vi "CONEX_FUNCTIONAL_GLOBAL.vi"(6 "Axis":enum16{"X", "Y", "Z", "XY", "XZ", "YZ", "XYZ"}(ring), 8 "error in":errorcluster, 9 "ASCII command":string, 10 "Position":dbl[](array[numeric]), 11 "Command":T1(ring)) -> (0 "error out":errorcluster, 1 "ASCII response":string[](array[string]), 2 "Current Position":dbl[](array[numeric]))   [LabVIEW 2013]
uses:
  <vilib>/Instr/_visa.llb/VISA Flush IO Buffer Mask.ctl
  <vilib>/Instr/_visa.llb/VISA Configure Serial Port (Instr).vi
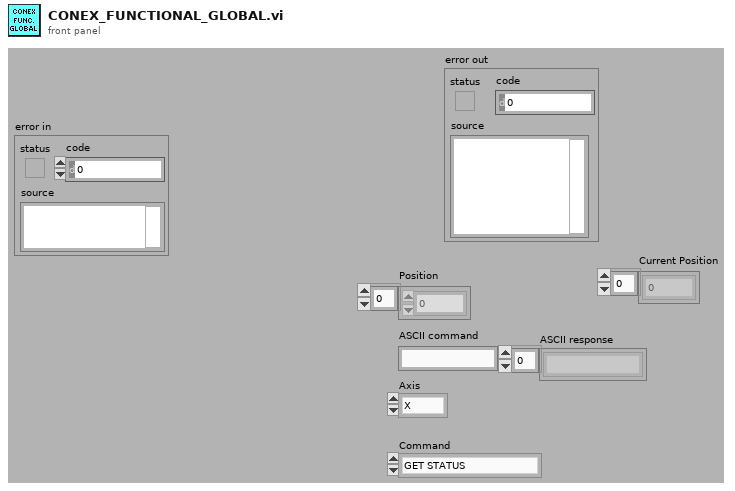
[diagram p1: front panel]
types:
  T1 = enum16{"GET STATUS", "ABS MOVE", "GET POS", "REL MOVE", "INIT", "CLOSE", "HOME", "READ ASCII", "ASCII", "SET ULIM", "STOP", "SET LLIM"}
  T2 = typedef "VISA Flush IO Buffer Mask.ctl" = u16
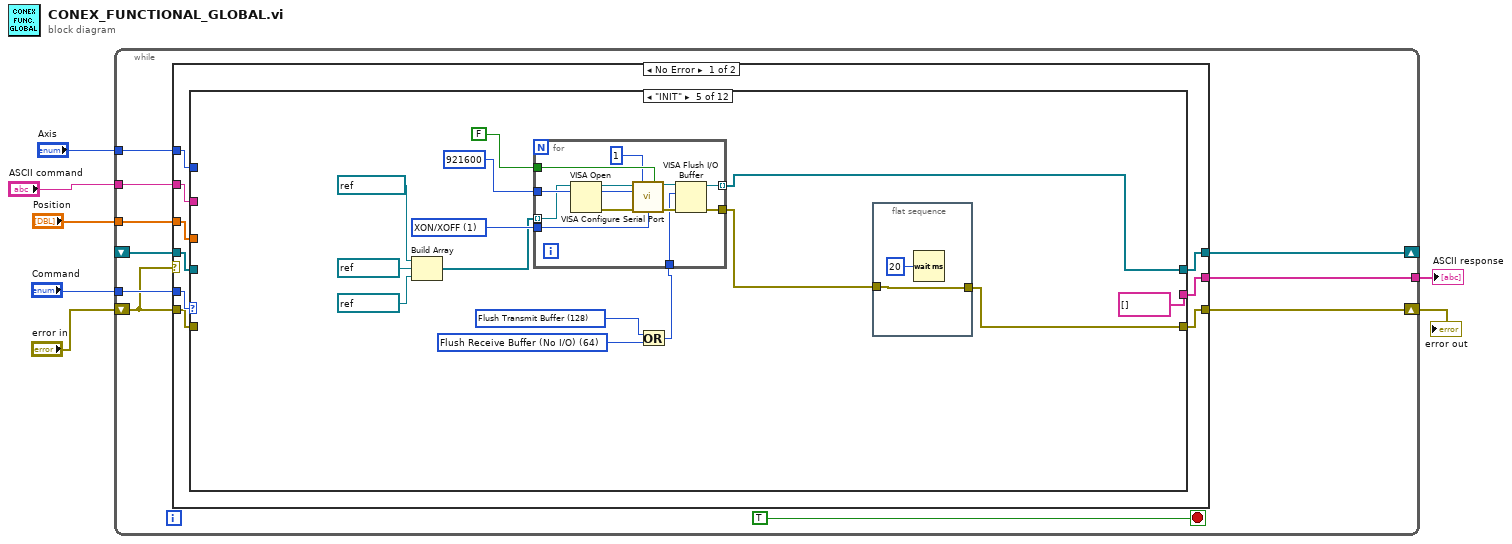
[diagram p0: block diagram]
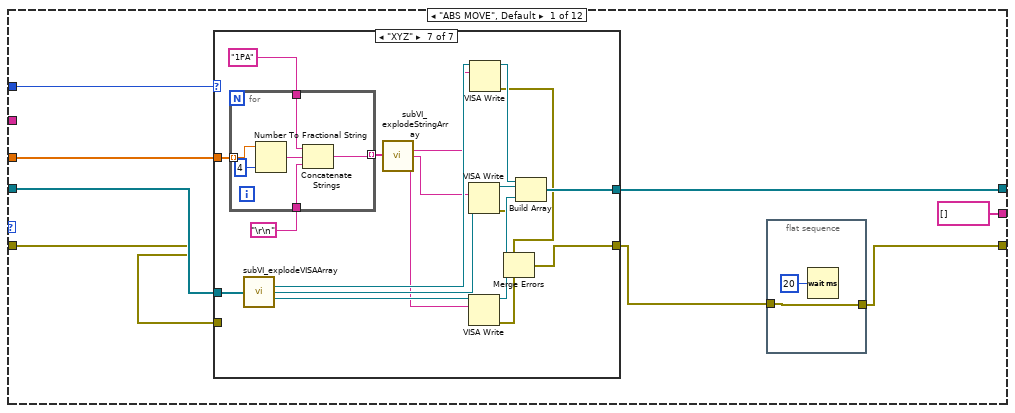
[diagram p2: hidden frame]
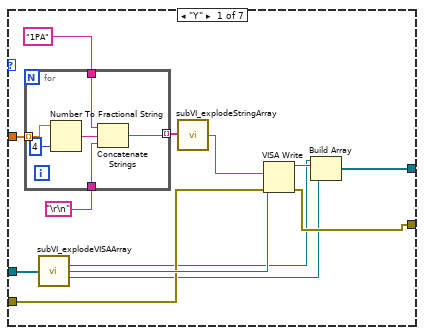
[diagram p3: hidden frame]
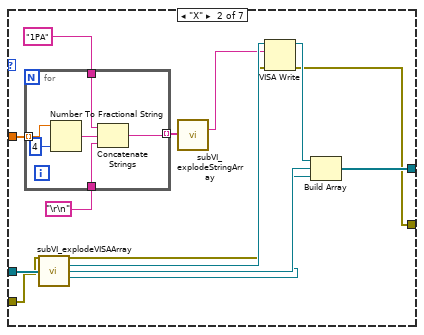
[diagram p4: hidden frame]
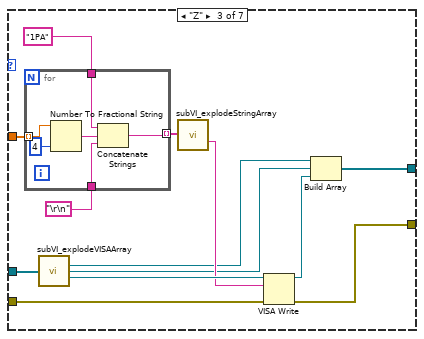
[diagram p5: hidden frame]
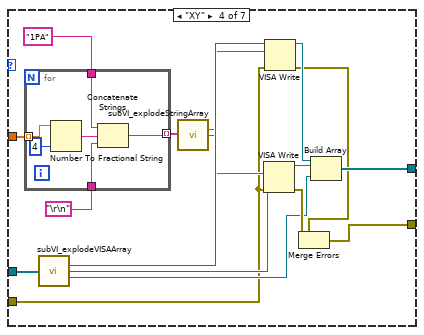
[diagram p6: hidden frame]
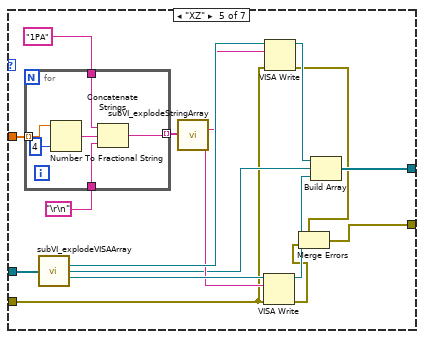
[diagram p7: hidden frame]
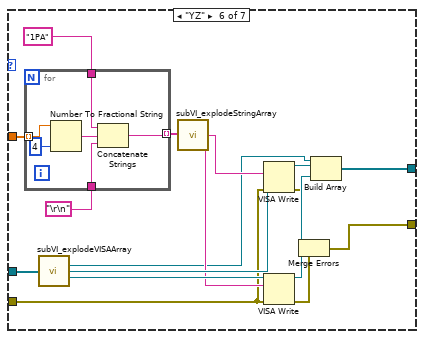
[diagram p8: hidden frame]
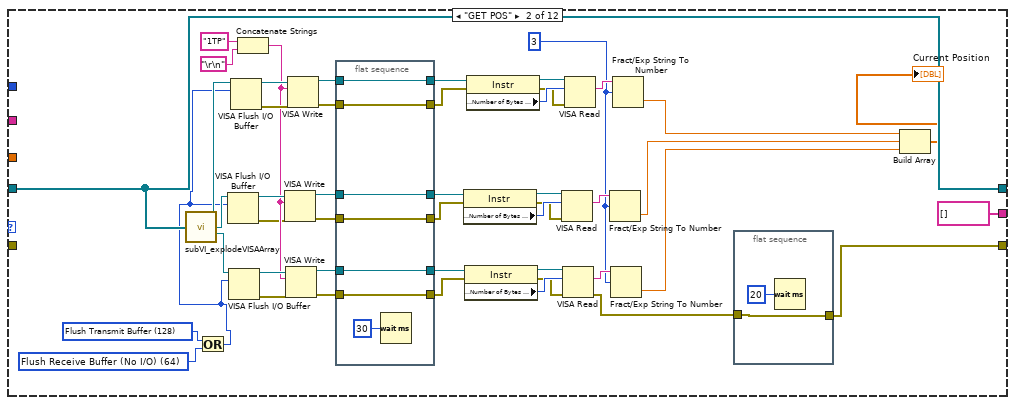
[diagram p9: hidden frame]
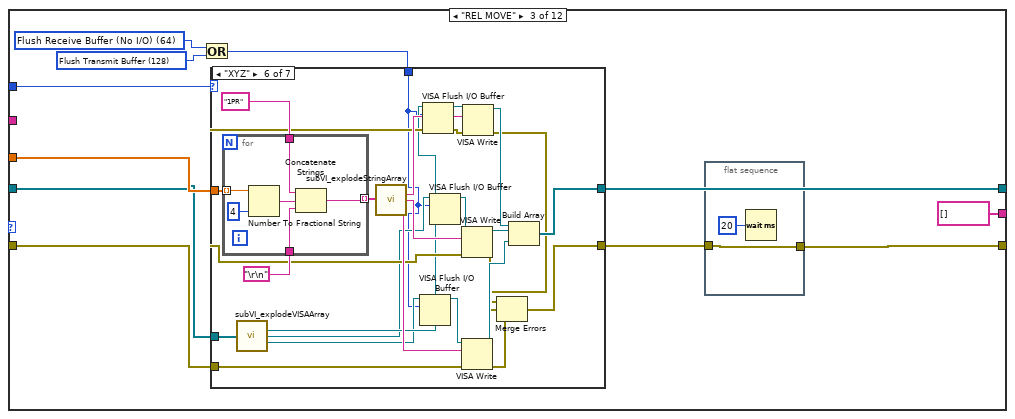
[diagram p10: hidden frame]
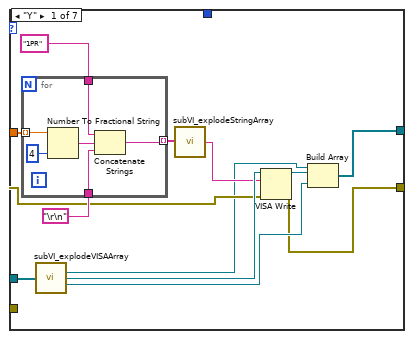
[diagram p11: hidden frame]
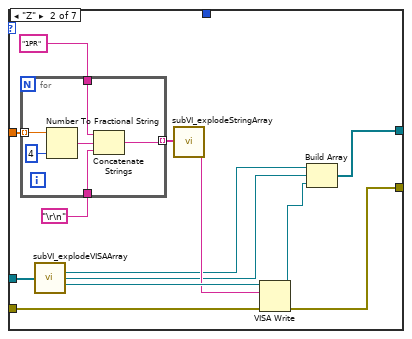
[diagram p12: hidden frame]
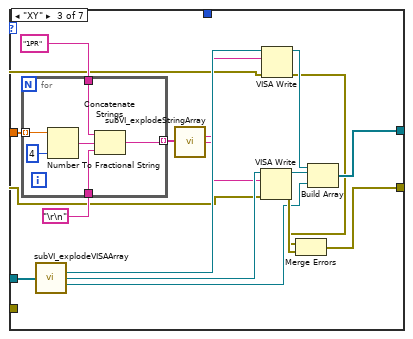
[diagram p13: hidden frame]
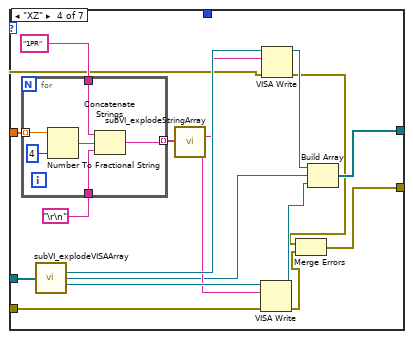
[diagram p14: hidden frame]
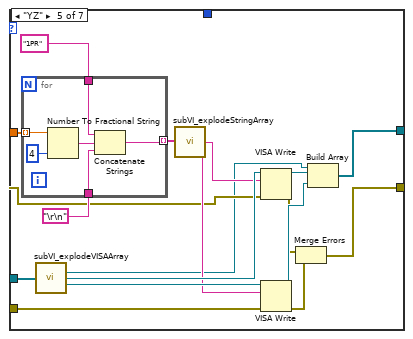
[diagram p15: hidden frame]
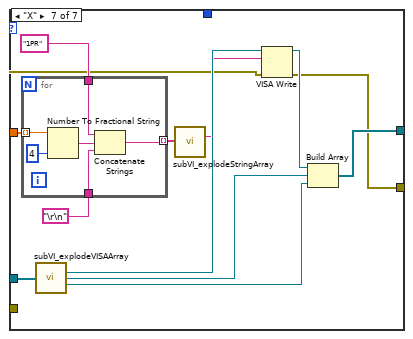
[diagram p16: hidden frame]
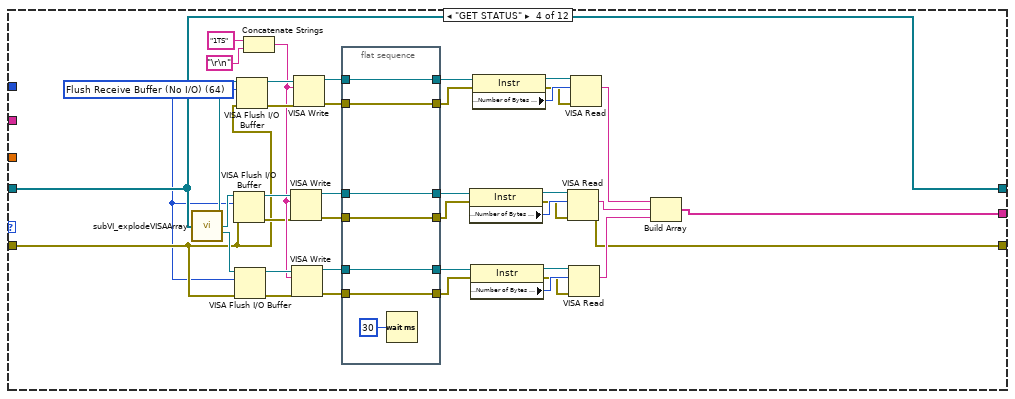
[diagram p17: hidden frame]
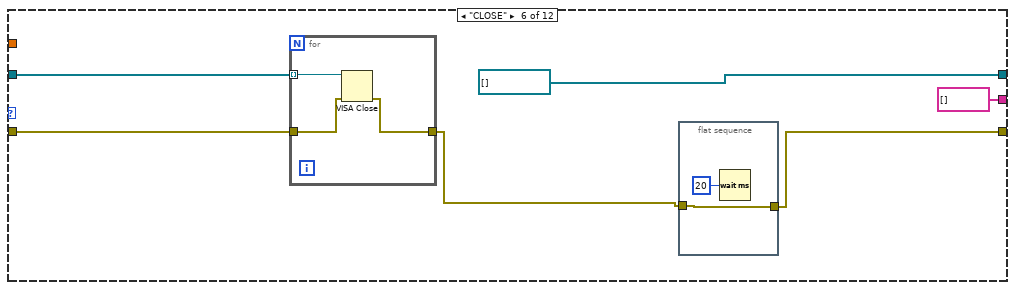
[diagram p18: hidden frame]
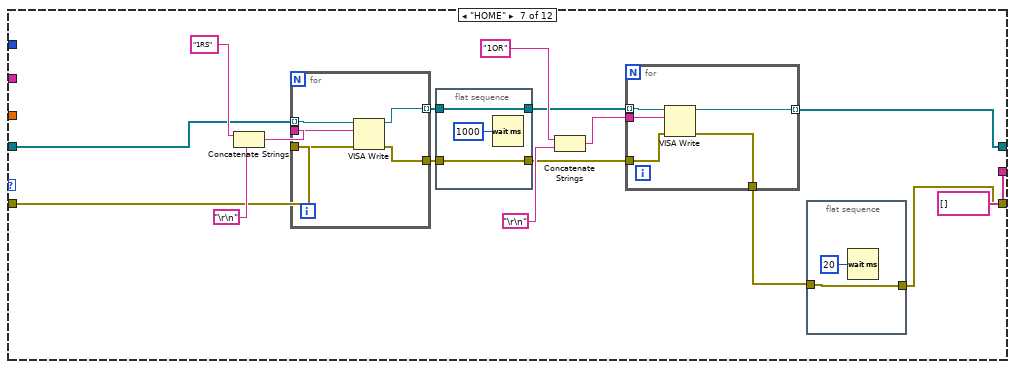
[diagram p19: hidden frame]
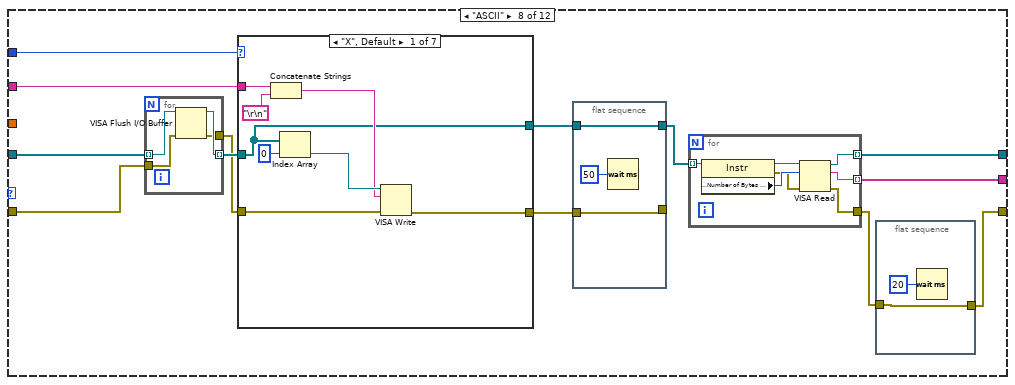
[diagram p20: hidden frame]
diagram:
  n1 = while {
    tunnel: "Command" -> [w17]
    shift-right: [w16] -> _
    shift-left: _ -> [w14]
    shift-right: [w15] -> w3
    shift-left: "error in" -> [w8]
    tunnel: "Position" -> [w13]
    tunnel: "ASCII command" -> [w11]
    tunnel: "Axis" -> [w10]
    tunnel: [w9] -> w1
    stop <- TRUE stop-if-true
    n2 = case shown="No Error" w8 {
      tunnel: w17 -> [w26 _]
      tunnel: [w25 refnum<visa-resource-name>[] []] -> w16
      tunnel: [w24 errorcluster {"status"=FALSE, "code"=0, "source"=""} ("error out")] -> w15
      tunnel: w14 -> [w23 w812]
      tunnel: w8 -> [w22 w811]
      tunnel: w13 -> [w21 _]
      tunnel: w11 -> [w20 _]
      tunnel: w10 -> [w19 _]
      tunnel: [w18 string[] []] -> w9
      frame No Error {
        n3 = case shown="\"INIT\"" w26 {
          tunnel: [w32 w232 w252 w417 w474 refnum<visa-resource-name>[] [] w513 w535 w638 w653 w671 w690] -> w25
          tunnel: [w27 w188 w245 w415 w462 w490 w501 w532 w635 w651 w669 w687] -> w24
          tunnel: w23 -> [w34 w232 w253 w417 _ w495 w509 w540 w643 w654 w672 w693]
          tunnel: w22 -> [w30 _ w254 w416 _ w494 w508 w538 w639 w657 w675 w692]
          tunnel: w21 -> [w33 _ w255 _ _ _ _ _ _ w655 w673 _]
          tunnel: w20 -> [_ _ _ _ _ _ _ w543 _ _ _ w694]
          tunnel: w19 -> [w31 _ w251 _ _ _ _ w544 _ _ _ w691]
          tunnel: [string[] [] string[] [] string[] [] w418 string[] [] string[] [] string[] [] w534 string[] [] string[] [] string[] [] w689] -> w18
          frame "ABS MOVE", Default {
            n4 = case shown="\"XYZ\"" w31 {
              tunnel: w34 -> [w49 w68 w87 w110 w133 w156 w181]
              tunnel: w33 -> [w47 w66 w85 w107 w130 w153 w177]
              tunnel: [w41 w60 w79 w99 w122 w145 w167] -> w32
              tunnel: [w40 w57 w76 w96 w120 w142 w163] -> w28
              tunnel: w30 -> [w39 w56 w75 w94 w118 w140 _]
              frame "Y" {
                n5 = for {
                  tunnel: w47 -> [w55] mode=indexing
                  tunnel: "1PA" -> [w53]
                  tunnel: "\r\n" -> [w52]
                  tunnel: [w51] -> w44 mode=indexing
                  n6 = Number To Fractional String(number=w55, precision (6)=i16 4) -> (F-format string=w54:string)  [unwired: 2 in]
                  n7 = Concatenate Strings(w53, w54, w52) -> (w51:string)
                }
                n8 = call "subVI_explodeVISAArray.vi"("Array"=w49) -> ("x"=w38:refnum<visa-resource-name>, "y"=w48:refnum<visa-resource-name>, "z"=w37:refnum<visa-resource-name>)  [unwired: 12 in]
                n9 = call "subVI_explodeStringArray.vi"("Array"=w44) -> ("y"=w43:string)  [unwired: 12 in, 2 out]
                n10 = VISA Write(VISA resource name=w48, write buffer=w43, error in (no error)=w39) -> (VISA resource name out=w42:refnum<visa-resource-name>, error out=w40:errorcluster)  [unwired: 1 out]
                n11 = Build Array(w38, w42, w37) -> (w41:refnum<visa-resource-name>[])
              }
              frame "X" {
                n12 = for {
                  tunnel: w66 -> [w74] mode=indexing
                  tunnel: "1PA" -> [w72]
                  tunnel: "\r\n" -> [w71]
                  tunnel: [w70] -> w63 mode=indexing
                  n13 = Number To Fractional String(number=w74, precision (6)=i16 4) -> (F-format string=w73:string)  [unwired: 2 in]
                  n14 = Concatenate Strings(w72, w73, w71) -> (w70:string)
                }
                n15 = call "subVI_explodeVISAArray.vi"("Array"=w68) -> ("x"=w67:refnum<visa-resource-name>, "y"=w59:refnum<visa-resource-name>, "z"=w58:refnum<visa-resource-name>)  [unwired: 12 in]
                n16 = call "subVI_explodeStringArray.vi"("Array"=w63) -> ("x"=w62:string)  [unwired: 12 in, 2 out]
                n17 = VISA Write(VISA resource name=w67, write buffer=w62, error in (no error)=w56) -> (VISA resource name out=w61:refnum<visa-resource-name>, error out=w57:errorcluster)  [unwired: 1 out]
                n18 = Build Array(w61, w59, w58) -> (w60:refnum<visa-resource-name>[])
              }
              frame "Z" {
                n19 = for {
                  tunnel: w85 -> [w93] mode=indexing
                  tunnel: "1PA" -> [w91]
                  tunnel: "\r\n" -> [w90]
                  tunnel: [w89] -> w82 mode=indexing
                  n20 = Number To Fractional String(number=w93, precision (6)=i16 4) -> (F-format string=w92:string)  [unwired: 2 in]
                  n21 = Concatenate Strings(w91, w92, w90) -> (w89:string)
                }
                n22 = call "subVI_explodeVISAArray.vi"("Array"=w87) -> ("x"=w78:refnum<visa-resource-name>, "y"=w77:refnum<visa-resource-name>, "z"=w86:refnum<visa-resource-name>)  [unwired: 12 in]
                n23 = call "subVI_explodeStringArray.vi"("Array"=w82) -> ("z"=w81:string)  [unwired: 12 in, 2 out]
                n24 = VISA Write(VISA resource name=w86, write buffer=w81, error in (no error)=w75) -> (VISA resource name out=w80:refnum<visa-resource-name>, error out=w76:errorcluster)  [unwired: 1 out]
                n25 = Build Array(w78, w77, w80) -> (w79:refnum<visa-resource-name>[])
              }
              frame "XY" {
                n26 = for {
                  tunnel: w107 -> [w116] mode=indexing
                  tunnel: "1PA" -> [w114]
                  tunnel: "\r\n" -> [w113]
                  tunnel: [w112] -> w104 mode=indexing
                  n27 = Number To Fractional String(number=w116, precision (6)=i16 4) -> (F-format string=w115:string)  [unwired: 2 in]
                  n28 = Concatenate Strings(w114, w115, w113) -> (w112:string)
                }
                n29 = call "subVI_explodeVISAArray.vi"("Array"=w110) -> ("x"=w109:refnum<visa-resource-name>, "y"=w108:refnum<visa-resource-name>, "z"=w95:refnum<visa-resource-name>)  [unwired: 12 in]
                n30 = call "subVI_explodeStringArray.vi"("Array"=w104) -> ("x"=w103:string, "y"=w102:string)  [unwired: 12 in, 1 out]
                n31 = VISA Write(VISA resource name=w108, write buffer=w102, error in (no error)=w94) -> (VISA resource name out=w100:refnum<visa-resource-name>, error out=w97:errorcluster)  [unwired: 1 out]
                n32 = VISA Write(VISA resource name=w109, write buffer=w103, error in (no error)=w94) -> (VISA resource name out=w101:refnum<visa-resource-name>, error out=w98:errorcluster)  [unwired: 1 out]
                n33 = Merge Errors(w98, w97) -> (w96:errorcluster)
                n34 = Build Array(w101, w100, w95) -> (w99:refnum<visa-resource-name>[])
              }
              frame "XZ" {
                n35 = for {
                  tunnel: w130 -> [w139] mode=indexing
                  tunnel: "1PA" -> [w137]
                  tunnel: "\r\n" -> [w136]
                  tunnel: [w135] -> w127 mode=indexing
                  n36 = Number To Fractional String(number=w139, precision (6)=i16 4) -> (F-format string=w138:string)  [unwired: 2 in]
                  n37 = Concatenate Strings(w137, w138, w136) -> (w135:string)
                }
                n38 = call "subVI_explodeVISAArray.vi"("Array"=w133) -> ("x"=w132:refnum<visa-resource-name>, "y"=w119:refnum<visa-resource-name>, "z"=w131:refnum<visa-resource-name>)  [unwired: 12 in]
                n39 = call "subVI_explodeStringArray.vi"("Array"=w127) -> ("x"=w126:string, "z"=w125:string)  [unwired: 12 in, 1 out]
                n40 = VISA Write(VISA resource name=w131, write buffer=w125, error in (no error)=w118) -> (VISA resource name out=w123:refnum<visa-resource-name>, error out=w117:errorcluster)  [unwired: 1 out]
                n41 = VISA Write(VISA resource name=w132, write buffer=w126, error in (no error)=w118) -> (VISA resource name out=w124:refnum<visa-resource-name>, error out=w121:errorcluster)  [unwired: 1 out]
                n42 = Merge Errors(w121, w117) -> (w120:errorcluster)
                n43 = Build Array(w124, w119, w123) -> (w122:refnum<visa-resource-name>[])
              }
              frame "YZ" {
                n44 = for {
                  tunnel: w153 -> [w162] mode=indexing
                  tunnel: "1PA" -> [w160]
                  tunnel: "\r\n" -> [w159]
                  tunnel: [w158] -> w150 mode=indexing
                  n45 = Number To Fractional String(number=w162, precision (6)=i16 4) -> (F-format string=w161:string)  [unwired: 2 in]
                  n46 = Concatenate Strings(w160, w161, w159) -> (w158:string)
                }
                n47 = call "subVI_explodeVISAArray.vi"("Array"=w156) -> ("x"=w141:refnum<visa-resource-name>, "y"=w155:refnum<visa-resource-name>, "z"=w154:refnum<visa-resource-name>)  [unwired: 12 in]
                n48 = call "subVI_explodeStringArray.vi"("Array"=w150) -> ("y"=w149:string, "z"=w148:string)  [unwired: 12 in, 1 out]
                n49 = VISA Write(VISA resource name=w155, write buffer=w149, error in (no error)=w140) -> (VISA resource name out=w146:refnum<visa-resource-name>, error out=w144:errorcluster)  [unwired: 1 out]
                n50 = VISA Write(VISA resource name=w154, write buffer=w148, error in (no error)=w140) -> (VISA resource name out=w147:refnum<visa-resource-name>, error out=w143:errorcluster)  [unwired: 1 out]
                n51 = Merge Errors(w144, w143) -> (w142:errorcluster)
                n52 = Build Array(w141, w146, w147) -> (w145:refnum<visa-resource-name>[])
              }
              frame "XYZ" {
                n53 = for {
                  tunnel: w177 -> [w187] mode=indexing
                  tunnel: "1PA" -> [w185]
                  tunnel: "\r\n" -> [w184]
                  tunnel: [w183] -> w174 mode=indexing
                  n54 = Number To Fractional String(number=w187, precision (6)=i16 4) -> (F-format string=w186:string)  [unwired: 2 in]
                  n55 = Concatenate Strings(w185, w186, w184) -> (w183:string)
                }
                n56 = call "subVI_explodeVISAArray.vi"("Array"=w181) -> ("x"=w180:refnum<visa-resource-name>, "y"=w179:refnum<visa-resource-name>, "z"=w178:refnum<visa-resource-name>)  [unwired: 12 in]
                n57 = call "subVI_explodeStringArray.vi"("Array"=w174) -> ("x"=w173:string, "y"=w172:string, "z"=w171:string)  [unwired: 12 in]
                n58 = VISA Write(VISA resource name=w179, write buffer=w172) -> (VISA resource name out=w168:refnum<visa-resource-name>, error out=w165:errorcluster)  [unwired: 1 in, 1 out]
                n59 = VISA Write(VISA resource name=w178, write buffer=w171) -> (VISA resource name out=w169:refnum<visa-resource-name>, error out=w164:errorcluster)  [unwired: 1 in, 1 out]
                n60 = VISA Write(VISA resource name=w180, write buffer=w173) -> (VISA resource name out=w170:refnum<visa-resource-name>, error out=w166:errorcluster)  [unwired: 1 in, 1 out]
                n61 = Merge Errors(w166, w165, w164) -> (w163:errorcluster)
                n62 = Build Array(w170, w168, w169) -> (w167:refnum<visa-resource-name>[])
              }
            }
            n63 = flat-sequence {
              tunnel: w28 -> [w36]
              tunnel: [w36] -> w27
              frame #0 {
                n64 = Wait (ms)(milliseconds to wait=u32 20) -> ()  [unwired: 1 out]
              }
            }
          }
          frame "GET POS" {
            w191 = T2 64 items=["Flush Receive Buffer"=16, "Write Transmit Buffer to Device"=32, "Flush Receive Buffer (No I/O)"=64, "Flush Transmit Buffer"=128] ("Mask")
            w192 = T2 128 items=["Flush Receive Buffer"=16, "Write Transmit Buffer to Device"=32, "Flush Receive Buffer (No I/O)"=64, "Flush Transmit Buffer"=128] ("Mask")
            w195 = 3 ("offset")
            n65 = call "subVI_explodeVISAArray.vi"("Array"=w232) -> ("x"=w230:refnum<visa-resource-name>, "y"=w220:refnum<visa-resource-name>, "z"=w218:refnum<visa-resource-name>)  [unwired: 12 in]
            n66 = Or(x=w192, y=w191) -> (x .or. y?=w190:T2)
            n67 = VISA Flush I/O Buffer(VISA resource name=w220, mask (16)=w190) -> (VISA resource name out=w219:refnum<visa-resource-name>, error out=w214:errorcluster)  [unwired: 1 in]
            n68 = VISA Flush I/O Buffer(VISA resource name=w218, mask (16)=w190) -> (VISA resource name out=w217:refnum<visa-resource-name>, error out=w215:errorcluster)  [unwired: 1 in]
            n69 = VISA Flush I/O Buffer(VISA resource name=w230, mask (16)=w190) -> (VISA resource name out=w228:refnum<visa-resource-name>, error out=w229:errorcluster)  [unwired: 1 in]
            n70 = Concatenate Strings("1TP" ("string"), "\r\n") -> (w216:string)
            n71 = VISA Write(VISA resource name=w219, write buffer=w216, error in (no error)=w214) -> (VISA resource name out=w213:refnum<visa-resource-name>, error out=w210:errorcluster)  [unwired: 1 out]
            n72 = VISA Write(VISA resource name=w217, write buffer=w216, error in (no error)=w215) -> (VISA resource name out=w212:refnum<visa-resource-name>, error out=w211:errorcluster)  [unwired: 1 out]
            n73 = VISA Write(VISA resource name=w228, write buffer=w216, error in (no error)=w229) -> (VISA resource name out=w227:refnum<visa-resource-name>, error out=w226:errorcluster)  [unwired: 1 out]
            n74 = flat-sequence {
              tunnel: w227 -> [w244]
              tunnel: w226 -> [w243]
              tunnel: [w244] -> w225
              tunnel: [w243] -> w224
              tunnel: w213 -> [w241]
              tunnel: w212 -> [w240]
              tunnel: w211 -> [w239]
              tunnel: w210 -> [w238]
              tunnel: [w241] -> w209
              tunnel: [w240] -> w208
              tunnel: [w239] -> w207
              tunnel: [w238] -> w206
              frame #0 {
                n75 = Wait (ms)(milliseconds to wait=u32 30) -> ()  [unwired: 1 out]
              }
            }
            n76 = property class="Instr"(reference=w209, error in=w206) -> (reference out=w205:refnum<visa-resource-name>, error out=w200:errorcluster, "Serial Settings:Number of Bytes at Serial Port"=w203:u32)
            n77 = property class="Instr"(reference=w208, error in=w207) -> (reference out=w204:refnum<visa-resource-name>, error out=w201:errorcluster, "Serial Settings:Number of Bytes at Serial Port"=w202:u32)
            n78 = property class="Instr"(reference=w225, error in=w224) -> (reference out=w223:refnum<visa-resource-name>, error out=w221:errorcluster, "Serial Settings:Number of Bytes at Serial Port"=w222:u32)
            n79 = VISA Read(VISA resource name=w205, byte count=w203, error in (no error)=w200) -> (read buffer=w199:string)  [unwired: 3 out]
            n80 = VISA Read(VISA resource name=w204, byte count=w202, error in (no error)=w201) -> (read buffer=w198:string, error out=w189:errorcluster)  [unwired: 2 out]
            n81 = VISA Read(VISA resource name=w223, byte count=w222, error in (no error)=w221) -> (read buffer=w233:string)  [unwired: 3 out]
            n82 = Fract/Exp String To Number(string=w199, offset=w195) -> (number=w197:dbl)  [unwired: 2 in, 1 out]
            n83 = Fract/Exp String To Number(string=w198, offset=w195) -> (number=w196:dbl)  [unwired: 2 in, 1 out]
            n84 = Fract/Exp String To Number(string=w233, offset=w195) -> (number=w231:dbl)  [unwired: 2 in, 1 out]
            n85 = flat-sequence {
              tunnel: w189 -> [w237]
              tunnel: [w237] -> w188
              frame #0 {
                n86 = Wait (ms)(milliseconds to wait=u32 20) -> ()  [unwired: 1 out]
              }
            }
            n87 = Build Array(w231, w197, w196) -> (→"Current Position":dbl[])
          }
          frame "REL MOVE" {
            w248 = T2 128 items=["Flush Receive Buffer"=16, "Write Transmit Buffer to Device"=32, "Flush Receive Buffer (No I/O)"=64, "Flush Transmit Buffer"=128] ("Mask")
            w249 = T2 64 items=["Flush Receive Buffer"=16, "Write Transmit Buffer to Device"=32, "Flush Receive Buffer (No I/O)"=64, "Flush Transmit Buffer"=128] ("Mask")
            n88 = Or(x=w249, y=w248) -> (x .or. y?=w247:T2)
            n89 = case shown="\"XYZ\"" w251 {
              tunnel: w255 -> [w264 w283 w302 w326 w347 w377 w401]
              tunnel: w254 -> [w263 w282 w301 w325 w346 w376 w400]
              tunnel: w253 -> [w262 w281 w300 w324 w345 w375 w399]
              tunnel: [w261 w280 w299 w323 w344 w374 w398] -> w252
              tunnel: [w258 w279 w298 w322 w343 w373 w397] -> w246
              tunnel: w247 -> [_ _ _ _ _ w365 _]
              frame "Y" {
                n90 = for {
                  tunnel: "1PR" -> [w275]
                  tunnel: "\r\n" -> [w274]
                  tunnel: [w273] -> w267 mode=indexing
                  tunnel: w264 -> [w271] mode=indexing
                  n91 = Number To Fractional String(number=w271, precision (6)=i16 4) -> (F-format string=w276:string)  [unwired: 2 in]
                  n92 = Concatenate Strings(w275, w276, w274) -> (w273:string)
                }
                n93 = call "subVI_explodeVISAArray.vi"("Array"=w262) -> ("x"=w260:refnum<visa-resource-name>, "y"=w270:refnum<visa-resource-name>, "z"=w259:refnum<visa-resource-name>)  [unwired: 12 in]
                n94 = call "subVI_explodeStringArray.vi"("Array"=w267) -> ("y"=w266:string)  [unwired: 12 in, 2 out]
                n95 = VISA Write(VISA resource name=w270, write buffer=w266, error in (no error)=w263) -> (VISA resource name out=w265:refnum<visa-resource-name>, error out=w258:errorcluster)  [unwired: 1 out]
                n96 = Build Array(w260, w265, w259) -> (w261:refnum<visa-resource-name>[])
              }
              frame "Z" {
                n97 = for {
                  tunnel: "1PR" -> [w294]
                  tunnel: "\r\n" -> [w293]
                  tunnel: [w292] -> w286 mode=indexing
                  tunnel: w283 -> [w290] mode=indexing
                  n98 = Number To Fractional String(number=w290, precision (6)=i16 4) -> (F-format string=w295:string)  [unwired: 2 in]
                  n99 = Concatenate Strings(w294, w295, w293) -> (w292:string)
                }
                n100 = call "subVI_explodeVISAArray.vi"("Array"=w281) -> ("x"=w278:refnum<visa-resource-name>, "y"=w277:refnum<visa-resource-name>, "z"=w289:refnum<visa-resource-name>)  [unwired: 12 in]
                n101 = call "subVI_explodeStringArray.vi"("Array"=w286) -> ("z"=w285:string)  [unwired: 12 in, 2 out]
                n102 = VISA Write(VISA resource name=w289, write buffer=w285, error in (no error)=w282) -> (VISA resource name out=w284:refnum<visa-resource-name>, error out=w279:errorcluster)  [unwired: 1 out]
                n103 = Build Array(w278, w277, w284) -> (w280:refnum<visa-resource-name>[])
              }
              frame "XY" {
                n104 = for {
                  tunnel: "1PR" -> [w317]
                  tunnel: "\r\n" -> [w316]
                  tunnel: [w315] -> w308 mode=indexing
                  tunnel: w302 -> [w313] mode=indexing
                  n105 = Number To Fractional String(number=w313, precision (6)=i16 4) -> (F-format string=w318:string)  [unwired: 2 in]
                  n106 = Concatenate Strings(w317, w318, w316) -> (w315:string)
                }
                n107 = call "subVI_explodeVISAArray.vi"("Array"=w300) -> ("x"=w312:refnum<visa-resource-name>, "y"=w311:refnum<visa-resource-name>, "z"=w296:refnum<visa-resource-name>)  [unwired: 12 in]
                n108 = call "subVI_explodeStringArray.vi"("Array"=w308) -> ("x"=w307:string, "y"=w306:string)  [unwired: 12 in, 1 out]
                n109 = VISA Write(VISA resource name=w311, write buffer=w306, error in (no error)=w301) -> (VISA resource name out=w304:refnum<visa-resource-name>, error out=w303:errorcluster)  [unwired: 1 out]
                n110 = VISA Write(VISA resource name=w312, write buffer=w307, error in (no error)=w301) -> (VISA resource name out=w305:refnum<visa-resource-name>, error out=w297:errorcluster)  [unwired: 1 out]
                n111 = Merge Errors(w297, w303) -> (w298:errorcluster)
                n112 = Build Array(w305, w304, w296) -> (w299:refnum<visa-resource-name>[])
              }
              frame "XZ" {
                n113 = for {
                  tunnel: "1PR" -> [w340]
                  tunnel: "\r\n" -> [w339]
                  tunnel: [w338] -> w331 mode=indexing
                  tunnel: w326 -> [w336] mode=indexing
                  n114 = Number To Fractional String(number=w336, precision (6)=i16 4) -> (F-format string=w341:string)  [unwired: 2 in]
                  n115 = Concatenate Strings(w340, w341, w339) -> (w338:string)
                }
                n116 = call "subVI_explodeVISAArray.vi"("Array"=w324) -> ("x"=w335:refnum<visa-resource-name>, "y"=w319:refnum<visa-resource-name>, "z"=w334:refnum<visa-resource-name>)  [unwired: 12 in]
                n117 = call "subVI_explodeStringArray.vi"("Array"=w331) -> ("x"=w330:string, "z"=w329:string)  [unwired: 12 in, 1 out]
                n118 = VISA Write(VISA resource name=w334, write buffer=w329, error in (no error)=w325) -> (VISA resource name out=w327:refnum<visa-resource-name>, error out=w320:errorcluster)  [unwired: 1 out]
                n119 = VISA Write(VISA resource name=w335, write buffer=w330, error in (no error)=w325) -> (VISA resource name out=w328:refnum<visa-resource-name>, error out=w321:errorcluster)  [unwired: 1 out]
                n120 = Merge Errors(w321, w320) -> (w322:errorcluster)
                n121 = Build Array(w328, w319, w327) -> (w323:refnum<visa-resource-name>[])
              }
              frame "YZ" {
                n122 = for {
                  tunnel: "1PR" -> [w363]
                  tunnel: "\r\n" -> [w362]
                  tunnel: [w361] -> w354 mode=indexing
                  tunnel: w347 -> [w359] mode=indexing
                  n123 = Number To Fractional String(number=w359, precision (6)=i16 4) -> (F-format string=w364:string)  [unwired: 2 in]
                  n124 = Concatenate Strings(w363, w364, w362) -> (w361:string)
                }
                n125 = call "subVI_explodeVISAArray.vi"("Array"=w345) -> ("x"=w342:refnum<visa-resource-name>, "y"=w358:refnum<visa-resource-name>, "z"=w357:refnum<visa-resource-name>)  [unwired: 12 in]
                n126 = call "subVI_explodeStringArray.vi"("Array"=w354) -> ("y"=w353:string, "z"=w352:string)  [unwired: 12 in, 1 out]
                n127 = VISA Write(VISA resource name=w358, write buffer=w353, error in (no error)=w346) -> (VISA resource name out=w350:refnum<visa-resource-name>, error out=w349:errorcluster)  [unwired: 1 out]
                n128 = VISA Write(VISA resource name=w357, write buffer=w352, error in (no error)=w346) -> (VISA resource name out=w351:refnum<visa-resource-name>, error out=w348:errorcluster)  [unwired: 1 out]
                n129 = Merge Errors(w349, w348) -> (w343:errorcluster)
                n130 = Build Array(w342, w350, w351) -> (w344:refnum<visa-resource-name>[])
              }
              frame "XYZ" {
                n131 = for {
                  tunnel: "1PR" -> [w393]
                  tunnel: "\r\n" -> [w392]
                  tunnel: [w391] -> w386 mode=indexing
                  tunnel: w377 -> [w389] mode=indexing
                  n132 = Number To Fractional String(number=w389, precision (6)=i16 4) -> (F-format string=w394:string)  [unwired: 2 in]
                  n133 = Concatenate Strings(w393, w394, w392) -> (w391:string)
                }
                n134 = call "subVI_explodeVISAArray.vi"("Array"=w375) -> ("x"=w371:refnum<visa-resource-name>, "y"=w369:refnum<visa-resource-name>, "z"=w368:refnum<visa-resource-name>)  [unwired: 12 in]
                n135 = call "subVI_explodeStringArray.vi"("Array"=w386) -> ("x"=w385:string, "y"=w384:string, "z"=w383:string)  [unwired: 12 in]
                n136 = VISA Flush I/O Buffer(VISA resource name=w368, mask (16)=w365) -> (VISA resource name out=w367:refnum<visa-resource-name>)  [unwired: 1 in, 1 out]
                n137 = VISA Flush I/O Buffer(VISA resource name=w371, mask (16)=w365) -> (VISA resource name out=w370:refnum<visa-resource-name>)  [unwired: 1 in, 1 out]
                n138 = VISA Flush I/O Buffer(VISA resource name=w369, mask (16)=w365) -> (VISA resource name out=w366:refnum<visa-resource-name>)  [unwired: 1 in, 1 out]
                n139 = VISA Write(VISA resource name=w366, write buffer=w384, error in (no error)=w376) -> (VISA resource name out=w380:refnum<visa-resource-name>, error out=w379:errorcluster)  [unwired: 1 out]
                n140 = VISA Write(VISA resource name=w367, write buffer=w383, error in (no error)=w376) -> (VISA resource name out=w381:refnum<visa-resource-name>, error out=w378:errorcluster)  [unwired: 1 out]
                n141 = VISA Write(VISA resource name=w370, write buffer=w385, error in (no error)=w376) -> (VISA resource name out=w382:refnum<visa-resource-name>, error out=w372:errorcluster)  [unwired: 1 out]
                n142 = Merge Errors(w372, w379, w378) -> (w373:errorcluster)
                n143 = Build Array(w382, w380, w381) -> (w374:refnum<visa-resource-name>[])
              }
              frame "X" {
                n144 = for {
                  tunnel: "1PR" -> [w412]
                  tunnel: "\r\n" -> [w411]
                  tunnel: [w410] -> w404 mode=indexing
                  tunnel: w401 -> [w408] mode=indexing
                  n145 = Number To Fractional String(number=w408, precision (6)=i16 4) -> (F-format string=w413:string)  [unwired: 2 in]
                  n146 = Concatenate Strings(w412, w413, w411) -> (w410:string)
                }
                n147 = call "subVI_explodeVISAArray.vi"("Array"=w399) -> ("x"=w407:refnum<visa-resource-name>, "y"=w396:refnum<visa-resource-name>, "z"=w395:refnum<visa-resource-name>)  [unwired: 12 in]
                n148 = call "subVI_explodeStringArray.vi"("Array"=w404) -> ("x"=w403:string)  [unwired: 12 in, 2 out]
                n149 = VISA Write(VISA resource name=w407, write buffer=w403, error in (no error)=w400) -> (VISA resource name out=w402:refnum<visa-resource-name>, error out=w397:errorcluster)  [unwired: 1 out]
                n150 = Build Array(w402, w396, w395) -> (w398:refnum<visa-resource-name>[])
              }
            }
            n151 = flat-sequence {
              tunnel: w246 -> [w257]
              tunnel: [w257] -> w245
              frame #0 {
                n152 = Wait (ms)(milliseconds to wait=u32 20) -> ()  [unwired: 1 out]
              }
            }
          }
          frame "GET STATUS" {
            w414 = T2 64 items=["Flush Receive Buffer"=16, "Write Transmit Buffer to Device"=32, "Flush Receive Buffer (No I/O)"=64, "Flush Transmit Buffer"=128] ("Mask")
            n153 = call "subVI_explodeVISAArray.vi"("Array"=w417) -> ("x"=w452:refnum<visa-resource-name>, "y"=w442:refnum<visa-resource-name>, "z"=w440:refnum<visa-resource-name>)  [unwired: 12 in]
            n154 = VISA Flush I/O Buffer(VISA resource name=w442, mask (16)=w414, error in (no error)=w416) -> (VISA resource name out=w441:refnum<visa-resource-name>, error out=w436:errorcluster)
            n155 = VISA Flush I/O Buffer(VISA resource name=w440, mask (16)=w414, error in (no error)=w416) -> (VISA resource name out=w439:refnum<visa-resource-name>, error out=w437:errorcluster)
            n156 = VISA Flush I/O Buffer(VISA resource name=w452, mask (16)=w414, error in (no error)=w416) -> (VISA resource name out=w450:refnum<visa-resource-name>, error out=w451:errorcluster)
            n157 = Concatenate Strings("1TS" ("string"), "\r\n") -> (w438:string)
            n158 = VISA Write(VISA resource name=w441, write buffer=w438, error in (no error)=w436) -> (VISA resource name out=w435:refnum<visa-resource-name>, error out=w432:errorcluster)  [unwired: 1 out]
            n159 = VISA Write(VISA resource name=w439, write buffer=w438, error in (no error)=w437) -> (VISA resource name out=w434:refnum<visa-resource-name>, error out=w433:errorcluster)  [unwired: 1 out]
            n160 = VISA Write(VISA resource name=w450, write buffer=w438, error in (no error)=w451) -> (VISA resource name out=w449:refnum<visa-resource-name>, error out=w448:errorcluster)  [unwired: 1 out]
            n161 = flat-sequence {
              tunnel: w449 -> [w461]
              tunnel: w448 -> [w460]
              tunnel: [w461] -> w447
              tunnel: [w460] -> w446
              tunnel: w435 -> [w458]
              tunnel: w434 -> [w457]
              tunnel: w433 -> [w456]
              tunnel: w432 -> [w455]
              tunnel: [w458] -> w431
              tunnel: [w457] -> w430
              tunnel: [w456] -> w429
              tunnel: [w455] -> w428
              frame #0 {
                n162 = Wait (ms)(milliseconds to wait=u32 30) -> ()  [unwired: 1 out]
              }
            }
            n163 = property class="Instr"(reference=w431, error in=w428) -> (reference out=w427:refnum<visa-resource-name>, error out=w422:errorcluster, "Serial Settings:Number of Bytes at Serial Port"=w425:u32)
            n164 = property class="Instr"(reference=w430, error in=w429) -> (reference out=w426:refnum<visa-resource-name>, error out=w423:errorcluster, "Serial Settings:Number of Bytes at Serial Port"=w424:u32)
            n165 = property class="Instr"(reference=w447, error in=w446) -> (reference out=w445:refnum<visa-resource-name>, error out=w443:errorcluster, "Serial Settings:Number of Bytes at Serial Port"=w444:u32)
            n166 = VISA Read(VISA resource name=w427, byte count=w425, error in (no error)=w422) -> (read buffer=w420:string, error out=w415:errorcluster)  [unwired: 2 out]
            n167 = VISA Read(VISA resource name=w426, byte count=w424, error in (no error)=w423) -> (read buffer=w419:string)  [unwired: 3 out]
            n168 = VISA Read(VISA resource name=w445, byte count=w444, error in (no error)=w443) -> (read buffer=w421:string)  [unwired: 3 out]
            n169 = Build Array(w421, w420, w419) -> (w418:string[])
          }
          frame "INIT" {
            w467 = T2 64 items=["Flush Receive Buffer"=16, "Write Transmit Buffer to Device"=32, "Flush Receive Buffer (No I/O)"=64, "Flush Transmit Buffer"=128] ("Mask")
            w468 = T2 128 items=["Flush Receive Buffer"=16, "Write Transmit Buffer to Device"=32, "Flush Receive Buffer (No I/O)"=64, "Flush Transmit Buffer"=128] ("Mask")
            w472 = u16 1 items=["None", "XON/XOFF", "RTS/CTS", "XON/XOFF & RTS/CTS", "DTR/DSR", "XON/XOFF & DTR/DSR"] ("flow control (0:none)")
            n170 = Build Array(refnum<visa-resource-name> "COM20" ("VISA resource name"), refnum<visa-resource-name> "COM3" ("VISA resource name"), refnum<visa-resource-name> "COM4" ("VISA resource name")) -> (w469:refnum<visa-resource-name>[])
            n171 = Or(x=w468, y=w467) -> (x .or. y?=w466:T2)
            n172 = for {
              tunnel: u32 921600 ("baud rate (9600)") -> [w488]
              tunnel: w472 -> [w487]
              tunnel: FALSE ("Enable Termination\nChar (T)") -> [w486]
              tunnel: w469 -> [w484] mode=indexing
              tunnel: [w481] -> w474 mode=indexing
              tunnel: [w480] -> w463
              tunnel: w466 -> [w478]
              n173 = VISA Open(VISA resource name=w484) -> (VISA resource name=w483:refnum<visa-resource-name>, error out=w489:errorcluster)  [unwired: 4 in]
              n174 = call-poly "VISA Configure Serial Port"("VISA resource name"=w483, "timeout (10sec)"=u32 1, "Enable Termination\nChar (T)"=w486, "baud rate (9600)"=w488, "error in (no error)"=w489, "flow control (0:none)"=w487) -> ("VISA resource name out"=w482:refnum<visa-resource-name>, "error out"=w485:errorcluster)  [unwired: 8 in]
              n175 = VISA Flush I/O Buffer(VISA resource name=w482, mask (16)=w478, error in (no error)=w485) -> (VISA resource name out=w481:refnum<visa-resource-name>, error out=w480:errorcluster)
            }
            n176 = flat-sequence {
              tunnel: w463 -> [w477]
              tunnel: [w477] -> w462
              frame #0 {
                n177 = Wait (ms)(milliseconds to wait=u32 20) -> ()  [unwired: 1 out]
              }
            }
          }
          frame "CLOSE" {
            n178 = for {
              tunnel: w495 -> [w500] mode=indexing
              tunnel: w494 -> [w499]
              tunnel: [w498] -> w491
              n179 = VISA Close(VISA resource name=w500, error in (no error)=w499) -> (error out=w498:errorcluster)
            }
            n180 = flat-sequence {
              tunnel: w491 -> [w497]
              tunnel: [w497] -> w490
              frame #0 {
                n181 = Wait (ms)(milliseconds to wait=u32 20) -> ()  [unwired: 1 out]
              }
            }
          }
          frame "HOME" {
            n182 = Concatenate Strings("1RS", "\r\n") -> (w510:string)
            n183 = for {
              tunnel: w510 -> [w526]
              tunnel: w509 -> [w525] mode=indexing
              tunnel: [w524] -> w507 mode=indexing
              tunnel: w508 -> [w523]
              tunnel: [w522] -> w505
              n184 = VISA Write(VISA resource name=w525, write buffer=w526, error in (no error)=w523) -> (VISA resource name out=w524:refnum<visa-resource-name>, error out=w522:errorcluster)  [unwired: 1 out]
            }
            n185 = flat-sequence {
              tunnel: [w521] -> w506
              tunnel: w507 -> [w521]
              tunnel: w505 -> [w520]
              tunnel: [w520] -> w504
              frame #0 {
                n186 = Wait (ms)(milliseconds to wait=u32 1000) -> ()  [unwired: 1 out]
              }
            }
            n187 = Concatenate Strings("1OR", "\r\n") -> (w514:string)
            n188 = for {
              tunnel: w514 -> [w531]
              tunnel: w506 -> [w530] mode=indexing
              tunnel: [w529] -> w513 mode=indexing
              tunnel: [w528] -> w502
              tunnel: w504 -> [w527]
              n189 = VISA Write(VISA resource name=w530, write buffer=w531, error in (no error)=w527) -> (VISA resource name out=w529:refnum<visa-resource-name>, error out=w528:errorcluster)  [unwired: 1 out]
            }
            n190 = flat-sequence {
              tunnel: w502 -> [w518]
              tunnel: [w518] -> w501
              frame #0 {
                n191 = Wait (ms)(milliseconds to wait=u32 20) -> ()  [unwired: 1 out]
              }
            }
          }
          frame "ASCII" {
            n192 = for {
              tunnel: w540 -> [w557] mode=indexing
              tunnel: [w556] -> w539 mode=indexing
              tunnel: w538 -> [w555]
              tunnel: [w554] -> w537
              n193 = VISA Flush I/O Buffer(VISA resource name=w557, error in (no error)=w555) -> (VISA resource name out=w556:refnum<visa-resource-name>, error out=w554:errorcluster)  [unwired: 1 in]
            }
            n194 = case shown="\"X\", Default" w544 {
              tunnel: w543 -> [w566 w572 w581 w593 w602 w614 w622]
              tunnel: w539 -> [w561 w571 w579 w588 w601 w610 w621]
              tunnel: w537 -> [w563 w569 w580 w594 w599 w609 _]
              tunnel: [w562 w570 w577 w585 w600 w611 w628] -> w541
              tunnel: [w561 w571 w579 w588 w601 w610 w621] -> w542
              frame "X", Default {
                n195 = Concatenate Strings(w566, "\r\n") -> (w564:string)
                n196 = Index Array(array=w561, index=0) -> (element=w567:refnum<visa-resource-name>)
                n197 = VISA Write(VISA resource name=w567, write buffer=w564, error in (no error)=w563) -> (error out=w562:errorcluster)  [unwired: 2 out]
              }
              frame "Y" {
                n198 = Concatenate Strings(w572, "\r\n") -> (w573:string)
                n199 = Index Array(array=w571, index=1) -> (element=w575:refnum<visa-resource-name>)
                n200 = VISA Write(VISA resource name=w575, write buffer=w573, error in (no error)=w569) -> (error out=w570:errorcluster)  [unwired: 2 out]
              }
              frame "Z" {
                n201 = Concatenate Strings(w581, "\r\n") -> (w582:string)
                n202 = Index Array(array=w579, index=2) -> (element=w578:refnum<visa-resource-name>)
                n203 = VISA Write(VISA resource name=w578, write buffer=w582, error in (no error)=w580) -> (error out=w577:errorcluster)  [unwired: 2 out]
              }
              frame "XY" {
                n204 = Concatenate Strings(w593, "\r\n") -> (w589:string)
                n205 = Index Array(array=w588, index=0) -> (element=w592:refnum<visa-resource-name>)
                n206 = Index Array(array=w588, index=1) -> (element=w590:refnum<visa-resource-name>)
                n207 = VISA Write(VISA resource name=w592, write buffer=w589, error in (no error)=w594) -> (error out=w587:errorcluster)  [unwired: 2 out]
                n208 = VISA Write(VISA resource name=w590, write buffer=w589, error in (no error)=w594) -> (error out=w586:errorcluster)  [unwired: 2 out]
                n209 = Merge Errors(w587, w586) -> (w585:errorcluster)
              }
              frame "XZ" {
                n210 = Concatenate Strings(w602, "\r\n") -> (w605:string)
                n211 = Index Array(array=w601, index=0) -> (element=w598:refnum<visa-resource-name>)
                n212 = Index Array(array=w601, index=2) -> (element=w597:refnum<visa-resource-name>)
                n213 = VISA Write(VISA resource name=w598, write buffer=w605, error in (no error)=w599) -> (error out=w604:errorcluster)  [unwired: 2 out]
                n214 = VISA Write(VISA resource name=w597, write buffer=w605, error in (no error)=w599) -> (error out=w603:errorcluster)  [unwired: 2 out]
                n215 = Merge Errors(w604, w603) -> (w600:errorcluster)
              }
              frame "YZ" {
                n216 = Concatenate Strings(w614, "\r\n") -> (w617:string)
                n217 = Index Array(array=w610, index=1) -> (element=w613:refnum<visa-resource-name>)
                n218 = Index Array(array=w610, index=2) -> (element=w612:refnum<visa-resource-name>)
                n219 = VISA Write(VISA resource name=w613, write buffer=w617, error in (no error)=w609) -> (error out=w616:errorcluster)  [unwired: 2 out]
                n220 = VISA Write(VISA resource name=w612, write buffer=w617, error in (no error)=w609) -> (error out=w615:errorcluster)  [unwired: 2 out]
                n221 = Merge Errors(w616, w615) -> (w611:errorcluster)
              }
              frame "XYZ" {
                n222 = Concatenate Strings(w622, "\r\n") -> (w623:string)
                n223 = Index Array(array=w621, index=2) -> (element=w624:refnum<visa-resource-name>)
                n224 = Index Array(array=w621, index=0) -> (element=w626:refnum<visa-resource-name>)
                n225 = Index Array(array=w621, index=1) -> (element=w625:refnum<visa-resource-name>)
                n226 = VISA Write(VISA resource name=w626, write buffer=w623) -> (error out=w631:errorcluster)  [unwired: 1 in, 2 out]
                n227 = VISA Write(VISA resource name=w625, write buffer=w623) -> (error out=w630:errorcluster)  [unwired: 1 in, 2 out]
                n228 = VISA Write(VISA resource name=w624, write buffer=w623) -> (error out=w629:errorcluster)  [unwired: 1 in, 2 out]
                n229 = Merge Errors(w631, w630, w629) -> (w628:errorcluster)
              }
            }
            n230 = flat-sequence {
              tunnel: w542 -> [w559]
              tunnel: w541 -> [w558]
              tunnel: [w559] -> w536
              tunnel: [w558] -> _
              frame #0 {
                n231 = Wait (ms)(milliseconds to wait=u32 50) -> ()  [unwired: 1 out]
              }
            }
            n232 = for {
              tunnel: w536 -> [w553] mode=indexing
              tunnel: [w551] -> w535 mode=indexing
              tunnel: [w549] -> w534 mode=indexing
              tunnel: [w547] -> w533
              n233 = property class="Instr"(reference=w553) -> (reference out=w552:refnum<visa-resource-name>, error out=w548:errorcluster, "Serial Settings:Number of Bytes at Serial Port"=w550:u32)  [unwired: 1 in]
              n234 = VISA Read(VISA resource name=w552, byte count=w550, error in (no error)=w548) -> (VISA resource name out=w551:refnum<visa-resource-name>, read buffer=w549:string, error out=w547:errorcluster)  [unwired: 1 out]
            }
            n235 = flat-sequence {
              tunnel: w533 -> [w546]
              tunnel: [w546] -> w532
              frame #0 {
                n236 = Wait (ms)(milliseconds to wait=u32 20) -> ()  [unwired: 1 out]
              }
            }
          }
          frame "STOP" {
            n237 = Concatenate Strings("1ST", "\r\n") -> (w640:string)
            n238 = for {
              tunnel: w643 -> [w650] mode=indexing
              tunnel: w640 -> [w649]
              tunnel: w639 -> [w648]
              tunnel: [w647] -> w636
              tunnel: [w646] -> w638 mode=indexing
              n239 = VISA Write(VISA resource name=w650, write buffer=w649, error in (no error)=w648) -> (VISA resource name out=w646:refnum<visa-resource-name>, error out=w647:errorcluster)  [unwired: 1 out]
            }
            n240 = flat-sequence {
              tunnel: w636 -> [w645]
              tunnel: [w645] -> w635
              frame #0 {
                n241 = Wait (ms)(milliseconds to wait=u32 20) -> ()  [unwired: 1 out]
              }
            }
          }
          frame "SET ULIM" {
            n242 = for {
              tunnel: w655 -> [w662] mode=indexing
              tunnel: w654 -> [w661] mode=indexing
              tunnel: [w660] -> w653 mode=indexing
              shift-right: [w667] -> w652
              shift-left: w657 -> [w668]
              n243 = Number To Fractional String(number=w662) -> (F-format string=w665:string)  [unwired: 3 in]
              n244 = Concatenate Strings("1SR", w665, "\r\n") -> (w663:string)
              n245 = VISA Write(VISA resource name=w661, write buffer=w663, error in (no error)=w668) -> (VISA resource name out=w660:refnum<visa-resource-name>, error out=w667:errorcluster)  [unwired: 1 out]
            }
            n246 = flat-sequence {
              tunnel: w652 -> [w659]
              tunnel: [w659] -> w651
              frame #0 {
                n247 = Wait (ms)(milliseconds to wait=u32 20) -> ()  [unwired: 1 out]
              }
            }
          }
          frame "SET LLIM" {
            n248 = for {
              tunnel: w673 -> [w680] mode=indexing
              tunnel: w672 -> [w679] mode=indexing
              tunnel: [w678] -> w671 mode=indexing
              shift-right: [w685] -> w670
              shift-left: w675 -> [w686]
              n249 = Number To Fractional String(number=w680) -> (F-format string=w683:string)  [unwired: 3 in]
              n250 = Concatenate Strings("1SL", w683, "\r\n") -> (w681:string)
              n251 = VISA Write(VISA resource name=w679, write buffer=w681, error in (no error)=w686) -> (VISA resource name out=w678:refnum<visa-resource-name>, error out=w685:errorcluster)  [unwired: 1 out]
            }
            n252 = flat-sequence {
              tunnel: w670 -> [w677]
              tunnel: [w677] -> w669
              frame #0 {
                n253 = Wait (ms)(milliseconds to wait=u32 20) -> ()  [unwired: 1 out]
              }
            }
          }
          frame "READ ASCII" {
            n254 = case shown="\"X\", Default" w691 {
              tunnel: w694 -> [_ _ _ _ _ _ _]
              tunnel: w693 -> [w708 w717 w731 _ _ w781 w806]
              tunnel: w692 -> [w698 w716 _ w739 w756 _ w789]
              tunnel: [w706 w709 w722 w737 w753 w771 w790] -> w688
              tunnel: [w702 w710 w726 w740 w761 w772 w791] -> w690
              tunnel: [w701 w711 w725 w742 w757 w773 w792] -> w689
              frame "X", Default {
                w700 = "" ("element")
                n255 = call "subVI_explodeVISAArray.vi"("Array"=w708) -> ("x"=w699:refnum<visa-resource-name>, "y"=w704:refnum<visa-resource-name>, "z"=w703:refnum<visa-resource-name>)  [unwired: 12 in]
                n256 = VISA Read(VISA resource name=w699, byte count=u32 256, error in (no error)=w698) -> (VISA resource name out=w705:refnum<visa-resource-name>, read buffer=w707:string, error out=w706:errorcluster)  [unwired: 1 out]
                n257 = Build Array(w707, w700, w700) -> (w701:string[])
                n258 = Build Array(w705, w704, w703) -> (w702:refnum<visa-resource-name>[])
              }
              frame "Y" {
                w712 = "" ("element")
                n259 = call "subVI_explodeVISAArray.vi"("Array"=w717) -> ("x"=w719:refnum<visa-resource-name>, "y"=w718:refnum<visa-resource-name>, "z"=w720:refnum<visa-resource-name>)  [unwired: 12 in]
                n260 = property class="Instr"(reference=w718, error in=w716) -> (reference out=w715:refnum<visa-resource-name>, error out=w709:errorcluster, "Serial Settings:Number of Bytes at Serial Port"=w721:u32)
                n261 = VISA Read(VISA resource name=w715, byte count=w721) -> (VISA resource name out=w714:refnum<visa-resource-name>, read buffer=w713:string)  [unwired: 1 in, 2 out]
                n262 = Build Array(w712, w713, w712) -> (w711:string[])
                n263 = Build Array(w719, w714, w720) -> (w710:refnum<visa-resource-name>[])
              }
              frame "Z" {
                w723 = "" ("element")
                n264 = call "subVI_explodeVISAArray.vi"("Array"=w731) -> ("x"=w729:refnum<visa-resource-name>, "y"=w728:refnum<visa-resource-name>, "z"=w730:refnum<visa-resource-name>)  [unwired: 12 in]
                n265 = property class="Instr"(reference=w730) -> (reference out=w733:refnum<visa-resource-name>, error out=w732:errorcluster, "Serial Settings:Number of Bytes at Serial Port"=w734:u32)  [unwired: 1 in]
                n266 = VISA Read(VISA resource name=w733, byte count=w734, error in (no error)=w732) -> (VISA resource name out=w727:refnum<visa-resource-name>, read buffer=w724:string, error out=w722:errorcluster)  [unwired: 1 out]
                n267 = Build Array(w723, w723, w724) -> (w725:string[])
                n268 = Build Array(w729, w728, w727) -> (w726:refnum<visa-resource-name>[])
              }
              frame "XY" {
                n269 = call "subVI_explodeVISAArray.vi"() -> ("x"=w752:refnum<visa-resource-name>, "y"=w745:refnum<visa-resource-name>, "z"=w746:refnum<visa-resource-name>)  [unwired: 13 in]
                n270 = property class="Instr"(reference=w752, error in=w739) -> (reference out=w750:refnum<visa-resource-name>, error out=w748:errorcluster, "Serial Settings:Number of Bytes at Serial Port"=w751:u32)
                n271 = property class="Instr"(reference=w745, error in=w739) -> (reference out=w743:refnum<visa-resource-name>, error out=w738:errorcluster, "Serial Settings:Number of Bytes at Serial Port"=w744:u32)
                n272 = VISA Read(VISA resource name=w743, byte count=w744, error in (no error)=w738) -> (VISA resource name out=w741:refnum<visa-resource-name>, read buffer=w736:string, error out=w737:errorcluster)  [unwired: 1 out]
                n273 = VISA Read(VISA resource name=w750, byte count=w751, error in (no error)=w748) -> (VISA resource name out=w747:refnum<visa-resource-name>, read buffer=w749:string)  [unwired: 2 out]
                n274 = Build Array(w749, "" ("element"), w736) -> (w742:string[])
                n275 = Build Array(w747, w741, w746) -> (w740:refnum<visa-resource-name>[])
              }
              frame "XZ" {
                n276 = call "subVI_explodeVISAArray.vi"() -> ("x"=w768:refnum<visa-resource-name>, "y"=w766:refnum<visa-resource-name>, "z"=w767:refnum<visa-resource-name>)  [unwired: 13 in]
                n277 = property class="Instr"(reference=w768, error in=w756) -> (reference out=w764:refnum<visa-resource-name>, error out=w755:errorcluster, "Serial Settings:Number of Bytes at Serial Port"=w769:u32)
                n278 = property class="Instr"(reference=w767, error in=w756) -> (reference out=w765:refnum<visa-resource-name>, error out=w754:errorcluster, "Serial Settings:Number of Bytes at Serial Port"=w770:u32)
                n279 = VISA Read(VISA resource name=w765, byte count=w770, error in (no error)=w754) -> (VISA resource name out=w762:refnum<visa-resource-name>, read buffer=w759:string, error out=w753:errorcluster)  [unwired: 1 out]
                n280 = VISA Read(VISA resource name=w764, byte count=w769, error in (no error)=w755) -> (VISA resource name out=w763:refnum<visa-resource-name>, read buffer=w760:string)  [unwired: 2 out]
                n281 = Build Array(w760, "" ("element"), w759) -> (w757:string[])
                n282 = Build Array(w763, w766, w762) -> (w761:refnum<visa-resource-name>[])
              }
              frame "YZ" {
                n283 = call "subVI_explodeVISAArray.vi"("Array"=w781) -> ("x"=w779:refnum<visa-resource-name>, "y"=w782:refnum<visa-resource-name>, "z"=w780:refnum<visa-resource-name>)  [unwired: 12 in]
                n284 = property class="Instr"(reference=w782) -> (reference out=w787:refnum<visa-resource-name>, error out=w786:errorcluster, "Serial Settings:Number of Bytes at Serial Port"=w788:u32)  [unwired: 1 in]
                n285 = property class="Instr"(reference=w780) -> (reference out=w784:refnum<visa-resource-name>, error out=w783:errorcluster, "Serial Settings:Number of Bytes at Serial Port"=w785:u32)  [unwired: 1 in]
                n286 = VISA Read(VISA resource name=w784, byte count=w785, error in (no error)=w783) -> (VISA resource name out=w777:refnum<visa-resource-name>, read buffer=w774:string, error out=w771:errorcluster)  [unwired: 1 out]
                n287 = VISA Read(VISA resource name=w787, byte count=w788, error in (no error)=w786) -> (VISA resource name out=w778:refnum<visa-resource-name>, read buffer=w775:string)  [unwired: 2 out]
                n288 = Build Array("" ("element"), w775, w774) -> (w773:string[])
                n289 = Build Array(w779, w778, w777) -> (w772:refnum<visa-resource-name>[])
              }
              frame "XYZ" {
                n290 = call "subVI_explodeVISAArray.vi"("Array"=w806) -> ("x"=w805:refnum<visa-resource-name>)  [unwired: 12 in, 2 out]
                n291 = property class="Instr"(reference=w805, error in=w789) -> (reference out=w804:refnum<visa-resource-name>, "Serial Settings:Number of Bytes at Serial Port"=w800:u32)  [unwired: 1 out]
                n292 = property class="Instr"(reference=w805, error in=w789) -> (reference out=w803:refnum<visa-resource-name>, "Serial Settings:Number of Bytes at Serial Port"=w801:u32)  [unwired: 1 out]
                n293 = property class="Instr"(reference=w805, error in=w789) -> (reference out=w802:refnum<visa-resource-name>, error out=w790:errorcluster, "Serial Settings:Number of Bytes at Serial Port"=w799:u32)
                n294 = VISA Read(VISA resource name=w803, byte count=w801) -> (VISA resource name out=w797:refnum<visa-resource-name>, read buffer=w794:string)  [unwired: 1 in, 2 out]
                n295 = VISA Read(VISA resource name=w802, byte count=w799) -> (VISA resource name out=w798:refnum<visa-resource-name>, read buffer=w793:string)  [unwired: 1 in, 2 out]
                n296 = VISA Read(VISA resource name=w804, byte count=w800) -> (VISA resource name out=w796:refnum<visa-resource-name>, read buffer=w795:string)  [unwired: 1 in, 2 out]
                n297 = Build Array(w795, w794, w793) -> (w792:string[])
                n298 = Build Array(w796, w797, w798) -> (w791:refnum<visa-resource-name>[])
              }
            }
            n299 = flat-sequence {
              tunnel: w688 -> [w696]
              tunnel: [w696] -> w687
              frame #0 {
                n300 = Wait (ms)(milliseconds to wait=u32 20) -> ()  [unwired: 1 out]
              }
            }
          }
        }
      }
      frame Error {
        n301 = for {
          tunnel: w812 -> [w815] mode=indexing
          tunnel: w811 -> [w814]
          tunnel: [w813] -> w808
          n302 = VISA Close(VISA resource name=w815, error in (no error)=w814) -> (error out=w813:errorcluster)
        }
        n303 = call <vilib>:"Simple Error Handler.vi"("error in (no error)"=w808) -> ()  [unwired: 4 in, 5 out]
      }
    }
  }
  "ASCII response" <- w1
  "error out" <- w3
